vi "Next Index.vi"(8 "error in (no error)":errorcluster, 11 "Config Manager in":refnum<class "Config Manager.lvclass">) -> (0 "error out":errorcluster, 1 "Index":i32, 2 "Add to End":bool, 3 "Config Manager out":refnum<class "Config Manager.lvclass">)   [LabVIEW 2020, in "CDM-Config.lvlib" / "Config Manager.lvclass"]
uses:
  Config Manager.lvclass
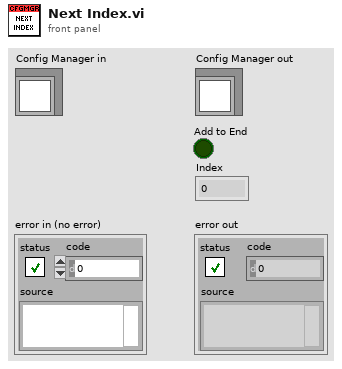
[diagram p1: front panel]
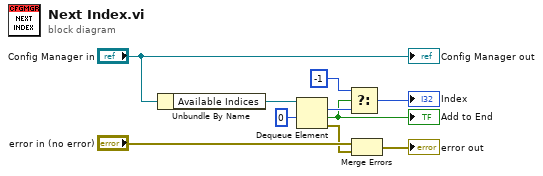
[diagram p0: block diagram]
diagram:
  n1 = Unbundle By Name("Config Manager in") -> ("Available Indices"=w8:refnum<queue>)
  n2 = Dequeue Element(queue=w8, timeout in ms (-1)=0) -> (element=w6:i32, timed out?=w5:bool, error out=w1:errorcluster)  [unwired: 1 in, 1 out]
  "Add to End" <- w5
  n3 = Select(t=-1, s=w5, f=w6) -> (s? t:f=→"Index":i32)
  n4 = Merge Errors("error in (no error)", w1) -> (→"error out":errorcluster)
  "Config Manager out" <- "Config Manager in"
